vi "NanotecSMCPD.reset axis position error.vi"(0 "i ref in":refnum<vi>, 1 "axis":i32, 3 "ms timeout (10000)":i32=10000, 5 "error in (no error)":errorcluster) -> (14 "i ref out":refnum<vi>, 19 "error out":errorcluster)   [LabVIEW 2014, in "NanotecSMCPD.lvlib"]
doc: "Resets the axis position error."
uses:
  NanotecSMCPD.lvlib
  CSCore/CSSystem/CoreDefs/CoreDefs.error_type.ctl
  CSCore/CSSystem/CoreDefs/CoreDefs.error_severity.ctl
  CSCore/CSApplicationBaseClasses/DeviceBase/DeviceBase.lvlib
  CSCore/CSSystem/CoreLib/CoreLib.lvlib
  CSCore/CSApplicationBaseClasses/MotorBase/MotorBase.lvlib
  CSinstr.lib/NanotecSMCPD/NanotecSMCPDDriver.lvlib
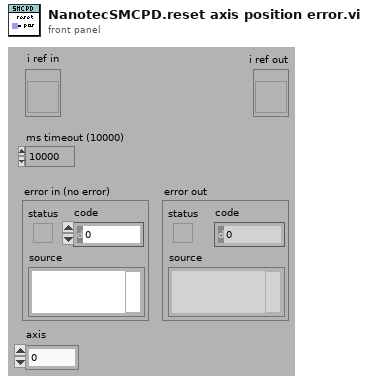
[diagram p1: front panel]
types:
  T1 = typedef "CoreDefs.error_severity.ctl" = enum16{"undefined", "information", "warning", "error", "fatal"}
  T2 = typedef "CoreDefs.error_type.ctl" = enum16{"no error", "can't load process", "can't unload process", "process does not exist", "can't install process", "can't remove process", "unknown function", "time out", "can't execute function", "duplicate queue name", "super not found", "caller queue invalid", "can't ping process", "unknown error", "VISA Error", "VISA timeout", "GPIB timeout", "GPIB error", "communication error", "data type mismatch", "can't read data from OPC server", "can't write data to OPC server", "OET error", "function not implemented", "process already exists", "invalid Shared Variable name", "error writing Shared Variable", "error reading Shared Variable", "invalid client name", "corrupt database", "unknown class", "call not authorized", "parameter out of range", "OET timeout: can't get data to modify", "invalid queue name", "requested operation incompatible with current state", "event undefined", "event disabled", "state undefined", "caller is not a friend", "EventBuilder: bad eventID", "EventBuilder: no DAQ devices", "a thread must not stop itself", "UNUSED ELEMENT4", "DiscArchiver: eventData incomplete", "DiscArchiver: eventData does not belong to run", "DiscArchiver: can't open file", "DiscArchiver: can't write to file", "DiscArchiver: available disc space low", "can't acquire semaphore", "error reading data from database", "notifier object is not existing", "can't register process", "can't unregister process", "illegal event type", "object disabled", "object already exists", "can't change state", "Instrument not found", "no connection to remote node", "invalid reference", "N/A", "UNUSED ELEMENT 1", "element not found", "illegal TCP/IP connection detected", "object does not exist", "invalid access ID", "unknown CS system", "invalid privilige", "unsupported data type", "unsupported server type", "IO server already exists", "Shared Variable already exists"}
  T3 = typedef "NanotecSMCPD.lvlib/NanotecSMCPD.i attribute.ctl" = cluster{"referencing":bool[], "stop":bool[], "AutoHalt ID":i32, "MethodQueue":refnum<queue>, "Referenced1Time?":bool[], "LastCommand ID":i32}
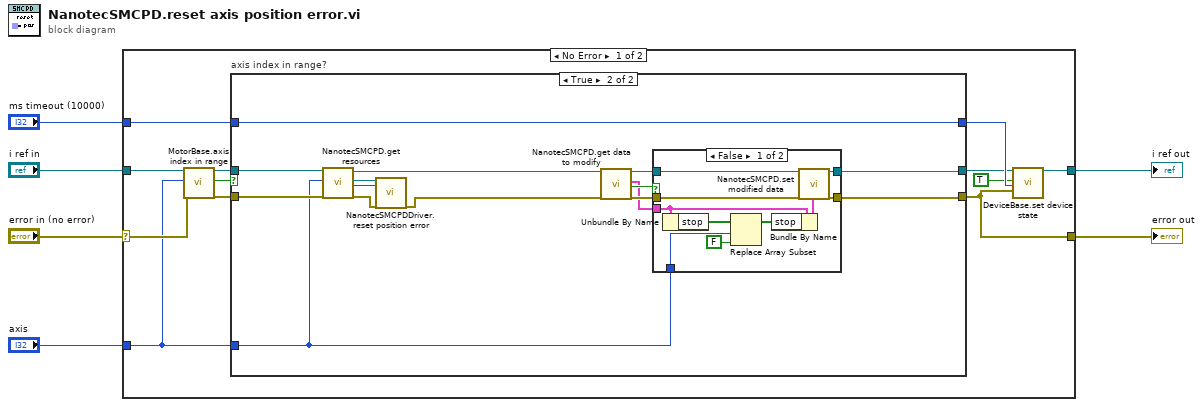
[diagram p0: block diagram]
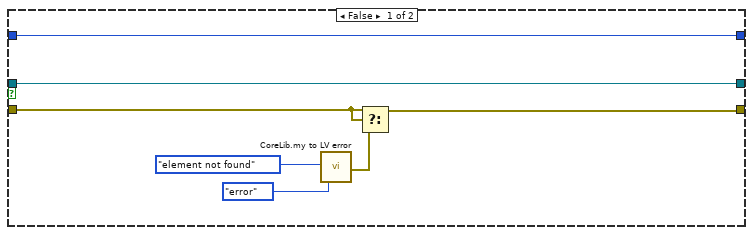
[diagram p2: hidden frame]
diagram:
  n1 = case shown="No Error" "error in (no error)" {
    selector: "error in (no error)" -> [w11 w53]
    tunnel: "ms timeout (10000)" -> [w8 _]
    tunnel: "i ref in" -> [w12 w54]
    tunnel: [w10 w53] -> w3
    tunnel: "axis" -> [w9 _]
    tunnel: [w7 w54] -> w1
    frame No Error {
      n2 = call "MotorBase.axis index in range.vi"("i ref in"=w12, "axisIndex"=w9, "error in (no error)"=w11) -> ("i ref out"=w16:refnum<vi>, "in range"=w15:bool, "error out"=w17:errorcluster)  [unwired: 14 in]
      n3 = case "axis index in range?" shown="True" w15 {
        tunnel: [w25 w28] -> w14
        tunnel: [w22 w27] -> w10
        tunnel: w8 -> [w19 w40]
        tunnel: w9 -> [_ w26]
        tunnel: w16 -> [w25 w39]
        tunnel: w17 -> [w23 w38]
        tunnel: [w19 w40] -> w18
        frame False {
          n4 = call "CoreLib.my to LV error.vi"("ErrorTypes"=CoreDefs.error_type."element not found", "severityLevel"=CoreDefs.error_severity."error") -> ("myErrorCluster"=w21:errorcluster)  [unwired: 16 in, 1 out]
          n5 = Select(t=w23, s=w23, f=w21) -> (s? t:f=w22:errorcluster)
        }
        frame True {
          n6 = call "NanotecSMCPD.get resources.vi"("i ref in"=w39, "axisNumber"=w26, "error in (no error)"=w38) -> ("i ref out"=w29:refnum<vi>, "VISA resource"=w37:refnum<visa-resource-name>, "address"=w36:i32, "error out"=w35:errorcluster)  [unwired: 13 in]
          n7 = call "NanotecSMCPDDriver.reset position error.vi"("VISA resource name"=w37, "contollerID"=w36, "error in (no error)"=w35) -> ("error out"=w30:errorcluster)  [unwired: 14 in, 2 out]
          n8 = call "NanotecSMCPD.get data to modify.vi"("i ref in"=w29, "error in (no error)"=w30) -> ("i ref out"=w33:refnum<vi>, "i attribute"=w31:T3, "timed out"=w34:bool, "error out"=w32:errorcluster)  [unwired: 14 in]
          n9 = case shown="False" w34 {
            tunnel: w33 -> [w50 w52]
            tunnel: [w49 w52] -> w28
            tunnel: w32 -> [w48 w51]
            tunnel: [w47 w51] -> w27
            tunnel: w31 -> [w46 _]
            tunnel: w26 -> [w42 _]
            frame False {
              n10 = Unbundle By Name(w46) -> ("stop"=w44:bool[])
              n11 = Replace Array Subset(array=w44, new element=FALSE ("new element/subarray"), index=w42) -> (w43:bool[])
              n12 = Bundle By Name(cluster=w46, "stop"=w43) -> (w45:T3)
              n13 = call "NanotecSMCPD.set modified data.vi"("i ref in"=w50, "i attribute"=w45, "error in (no error)"=w48) -> ("i ref out"=w49:refnum<vi>, "error out"=w47:errorcluster)  [unwired: 15 in]
            }
            frame True {
            }
          }
        }
      }
      n14 = call "DeviceBase.set device state.vi"("i ref in"=w14, "implicit"=TRUE, "ms timeout (10000)"=w18, "device error"=w10) -> ("i ref out"=w7:refnum<vi>)  [unwired: 13 in, 2 out]
    }
    frame Error {
    }
  }
  "error out" <- w3
  "i ref out" <- w1
